vi "3-8 Deocder_Working.vi"() -> ()   [LabVIEW 2012]
panel:
  in  "stop":bool
  out "Y7":bool
  out "Y6":bool
  out "Y5":bool
  out "Y4":bool
  out "Y3":bool
  out "Y2":bool
  out "Y1":bool
  out "Y0":bool
  in  "Boolean 3":bool
  in  "Boolean 2":bool
  in  "Boolean":bool
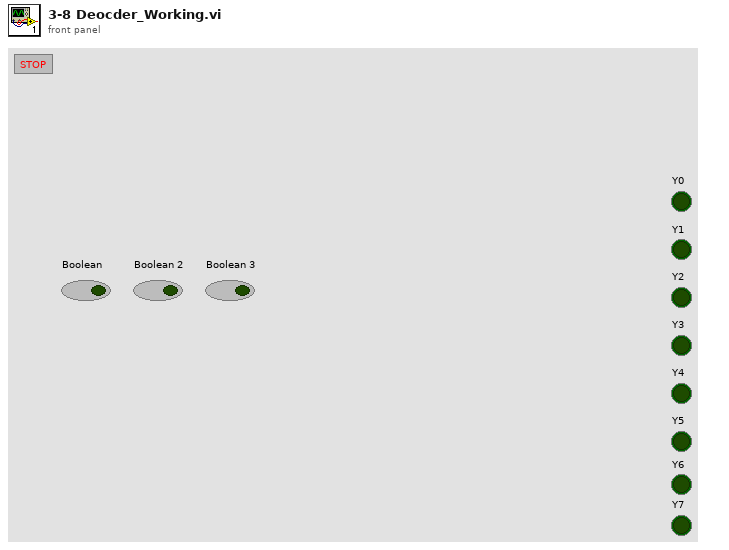
[diagram p1: front panel]
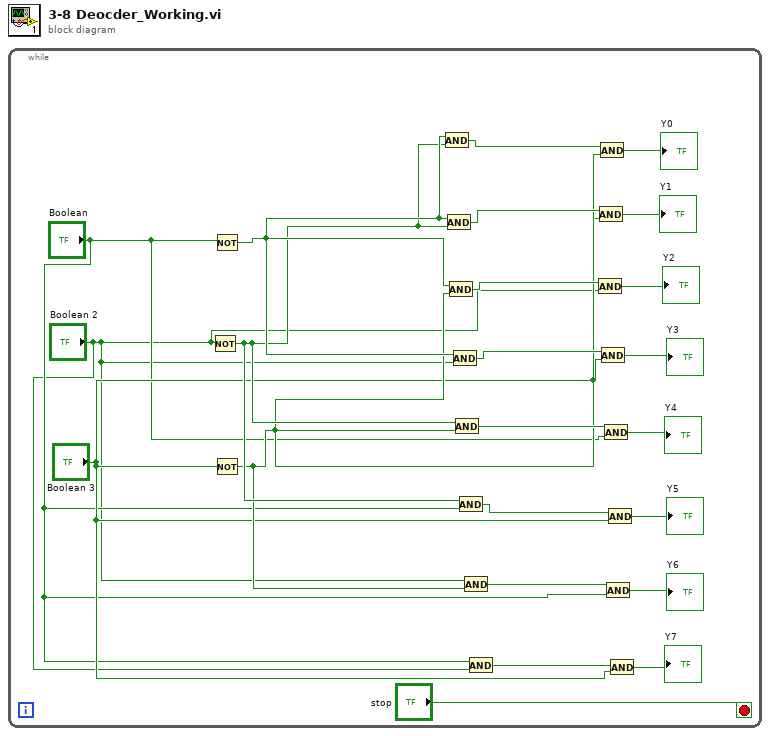
[diagram p0: block diagram]
diagram:
  n1 = while {
    stop <- "stop" stop-if-true
    n2 = Not(x="Boolean 2") -> (.not. x?=w6:bool)
    n3 = Not(x="Boolean") -> (.not. x?=w7:bool)
    n4 = Not(x="Boolean 3") -> (.not. x?=w5:bool)
    n5 = And(x=w7, y=w6) -> (x .and. y?=w15:bool)
    n6 = And(x=w7, y=w6) -> (x .and. y?=w14:bool)
    n7 = And(x=w7, y=w5) -> (x .and. y?=w13:bool)
    n8 = And(x=w7, y="Boolean 2") -> (x .and. y?=w12:bool)
    n9 = And(x=w6, y=w5) -> (x .and. y?=w11:bool)
    n10 = And(x=w6, y="Boolean") -> (x .and. y?=w10:bool)
    n11 = And(x="Boolean 2", y=w5) -> (x .and. y?=w9:bool)
    n12 = And(x="Boolean", y="Boolean 2") -> (x .and. y?=w8:bool)
    n13 = And(x=w13, y="Boolean 2") -> (x .and. y?=→"Y2":bool)
    n14 = And(x=w14, y="Boolean 3") -> (x .and. y?=→"Y1":bool)
    n15 = And(x=w15, y=w5) -> (x .and. y?=→"Y0":bool)
    n16 = And(x=w12, y="Boolean 3") -> (x .and. y?=→"Y3":bool)
    n17 = And(x=w11, y="Boolean") -> (x .and. y?=→"Y4":bool)
    n18 = And(x=w9, y="Boolean") -> (x .and. y?=→"Y6":bool)
    n19 = And(x=w10, y="Boolean 3") -> (x .and. y?=→"Y5":bool)
    n20 = And(x=w8, y="Boolean 3") -> (x .and. y?=→"Y7":bool)
  }
